vi "UploadUsers.vi"(8 "error in (no error)":errorcluster, 11 "DB in":refnum<class "DB.lvclass">) -> (0 "error out":errorcluster, 3 "DB out":refnum<class "DB.lvclass">)   [LabVIEW 2015, in "DB.lvclass"]
uses:
  DB.lvclass
  DB.lvclass/DB.ctl
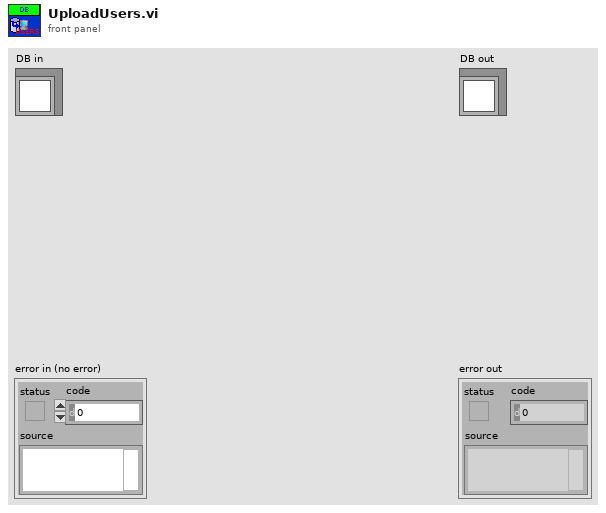
[diagram p1: front panel]
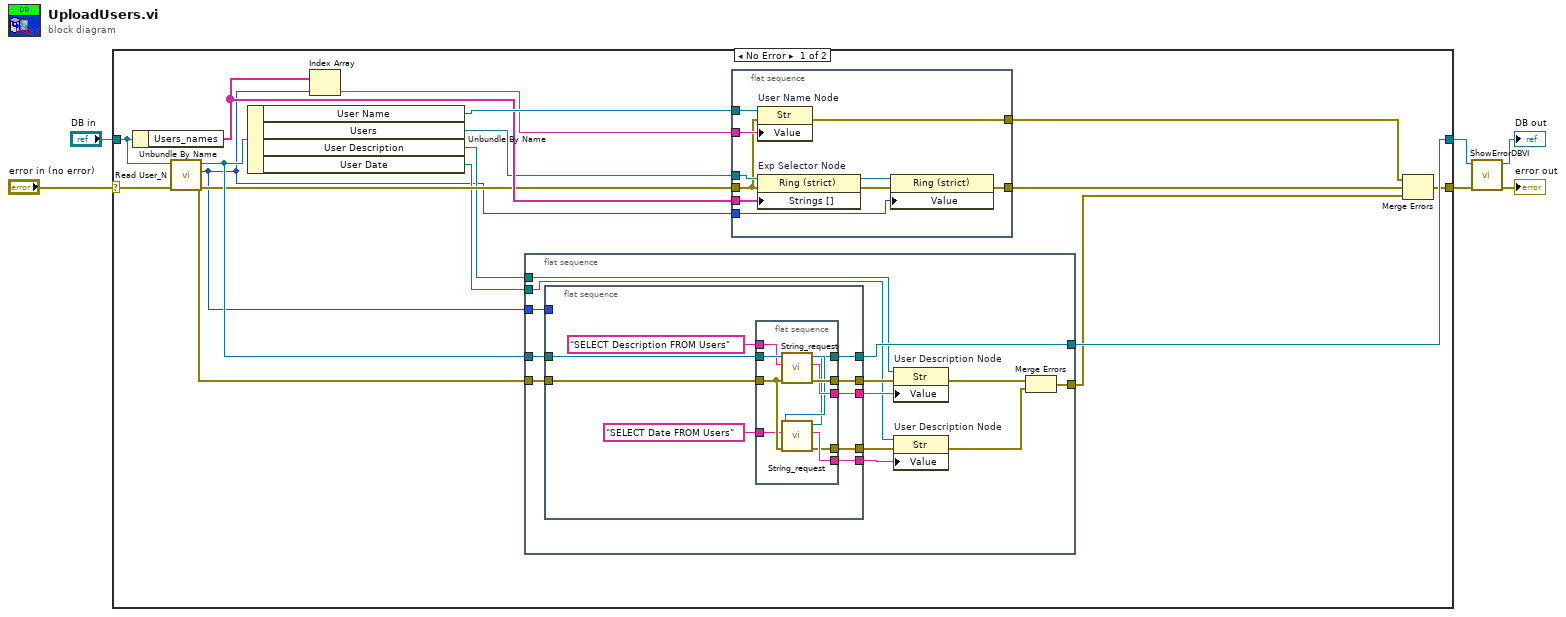
[diagram p0: block diagram]
diagram:
  n1 = case shown="No Error" "error in (no error)" {
    selector: "error in (no error)" -> [w21 w66]
    tunnel: [w14 w66] -> w6
    tunnel: [w15 w65] -> w5
    tunnel: "DB in" -> [w22 w65]
    frame No Error {
      n2 = Unbundle By Name(w22) -> ("Users_names"=w19:string[])
      n3 = call "Read User_N.vi"("error in (no error)"=w21, "DB in"=w22) -> ("error out"=w13:errorcluster, "Exp_N"=w7:i16, "DB out"=w16:refnum<class "DB.lvclass">)  [unwired: 7 in]
      n4 = Unbundle By Name(w16) -> ("User Name"=w20:refnum<vi>, "Users"=w18:refnum<vi>, "User Description"=w12:refnum<vi>, "User Date"=w8:refnum<vi>)
      n5 = Index Array(array=w19, index=w7) -> (element=w9:string)
      n6 = flat-sequence {
        tunnel: w16 -> [w35]
        tunnel: [w45] -> w15
        tunnel: w13 -> [w37]
        tunnel: w12 -> [w43]
        tunnel: [w39] -> w10
        tunnel: w8 -> [w41]
        tunnel: w7 -> [w34]
        frame #0 {
          n7 = flat-sequence {
            tunnel: [w54] -> w45
            tunnel: [w52] -> w44
            tunnel: [w51] -> w42
            tunnel: w37 -> [w50]
            tunnel: [w48] -> w36
            tunnel: w35 -> [w47]
            tunnel: w34 -> [_]
            tunnel: [w46] -> w33
            frame #0 {
              n8 = flat-sequence {
                tunnel: [w55] -> w54
                tunnel: "SELECT Description FROM Users" ("SQL request") -> [w58]
                tunnel: [w64] -> w52
                tunnel: [w63] -> w51
                tunnel: w50 -> [w62]
                tunnel: "SELECT Date FROM Users" ("SQL request") -> [w57]
                tunnel: [w61] -> w48
                tunnel: w47 -> [w60]
                tunnel: [w59] -> w46
                frame #0 {
                  n9 = call-dynamic "String_request.vi"("error in (no error)"=w62, "SQL request"=w58, "DB in"=w60) -> ("error out"=w64:errorcluster, "Result"=w63:string, "DB out"=w56:refnum<class "DB.lvclass">)  [unwired: 6 in]
                  n10 = call-dynamic "String_request.vi"("error in (no error)"=w62, "SQL request"=w57, "DB in"=w56) -> ("error out"=w59:errorcluster, "Result"=w61:string, "DB out"=w55:refnum<class "DB.lvclass">)  [unwired: 6 in]
                }
              }
            }
          }
          n11 = property on="User Description Node" class="Str"(reference=w43, error in=w44, "Value"=w42) -> (error out=w40:errorcluster)  [unwired: 1 out]
          n12 = property on="User Description Node" class="Str"(reference=w41, error in=w33, "Value"=w36) -> (error out=w38:errorcluster)  [unwired: 1 out]
          n13 = Merge Errors(w40, w38) -> (w39:errorcluster)
        }
      }
      n14 = flat-sequence {
        tunnel: w20 -> [w31]
        tunnel: w19 -> [w30]
        tunnel: w9 -> [w29]
        tunnel: w18 -> [w28]
        tunnel: [w27] -> w17
        tunnel: w7 -> [w25]
        tunnel: w13 -> [w24]
        tunnel: [w23] -> w11
        frame #0 {
          n15 = property on="User Name Node" class="Str"(reference=w31, error in=w24, "Value"=w29) -> (error out=w23:errorcluster)  [unwired: 1 out]
          n16 = property on="Exp Selector Node" class="Ring (strict)"(reference=w28, error in=w24, "Strings []"=w30) -> (reference out=w32:refnum<vi>, error out=w26:errorcluster)
          n17 = property class="Ring (strict)"(reference=w32, error in=w26, "Value"=w25) -> (error out=w27:errorcluster)  [unwired: 1 out]
        }
      }
      n18 = Merge Errors(w11, w17, w10) -> (w14:errorcluster)
    }
    frame Error {
    }
  }
  n19 = call "ShowErrorDBVI.vi"("error in (no error)"=w6, "DB in"=w5) -> ("error out"=→"error out":errorcluster, "DB out"=→"DB out":refnum<class "DB.lvclass">)  [unwired: 8 in]
